vi "Configure.vi"(8 "error in (no error)":errorcluster, 11 "StageSPIM in":refnum<class "StageSPIM.lvclass">) -> (0 "error out":errorcluster, 2 "cancelled?":bool, 3 "StageSPIM out":refnum<class "StageSPIM.lvclass">)   [LabVIEW 2012, in "StageSPIM.lvclass"]
doc: "The configure method configures the details for the RabbitMQ connection. \n\nIn the derived class, make a call to the parent for setting these parameters."
uses:
  StageSPIM.lvclass
  connection_type.ctl
  baud_rate_control.ctl
  port_control.ctl
  <vilib>/Utility/miscctls.llb/LVPointTypeDef.ctl
  StageSPIM.lvclass/StageSPIM.ctl
  <vilib>/Distrio/Murmex/Murmex/Murmex.lvclass
panel:
  in  "button::configure murmex":bool
  in  "button::ok":bool
  in  "button::cancel":bool
  in  "Tab Control":enum32{"Comport", "Stages", "Debug"}(tab)
  in  "Port":T1 items=["COM1", "COM2", "COM3", "COM4", "COM5", "COM6", "COM7", "COM8", "COM9", "COM10", "COM11", "COM12", "COM13", "COM14", "COM15", "COM16", "COM17", "COM18", "COM19", "COM20", "COM21", "COM22", "COM23", "COM24", "COM25", "COM26", "COM27", "COM28", "COM29", "COM30"]
  in  "Baudrate":T2=3 items=["9600", "14400", "19200", "38400", "57600", "115200"]
  in  "Interface":T3=enum."USB_DaisyChain"
  in  "S/N Master controller":string
  in  "Update frequency":dbl[unit]
  in  "speedFocus":dbl[unit]
  in  "speedZ":dbl[unit]
  in  "speedY":dbl[unit]
  in  "speedX":dbl[unit]
  in  "soft min limit":dbl[](array[numeric])
  in  "soft max limit":dbl[](array[numeric])
  # "startup speed"
  # "X"
  # "Y"
  # "Z"
  # "Focus"
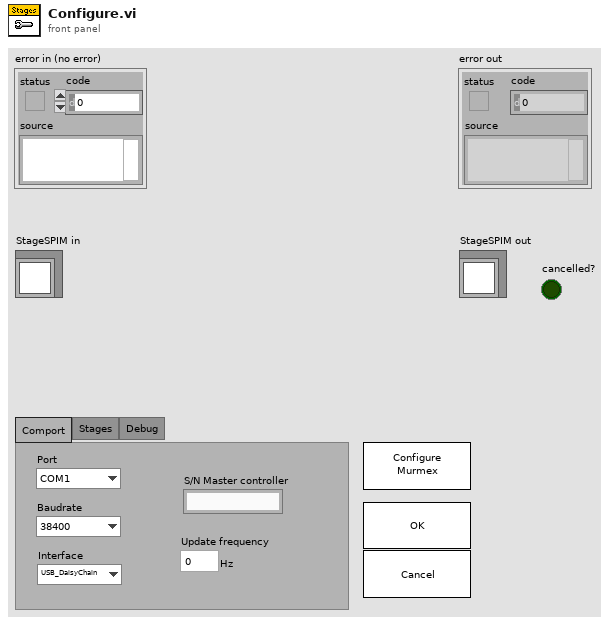
[diagram p1: front panel]
types:
  T1 = typedef "StageSPIM.lvclass/port_control.ctl" = i32
  T2 = typedef "StageSPIM.lvclass/baud_rate_control.ctl" = u16
  T3 = typedef "StageSPIM.lvclass/connection_type.ctl" = enum16{"RS232", "RS232 DaisyChain", "USB", "USB_DaisyChain"}
  T4 = typedef "LVPointTypeDef.ctl" = cluster{"Horizontal":i16, "Vertical":i16}
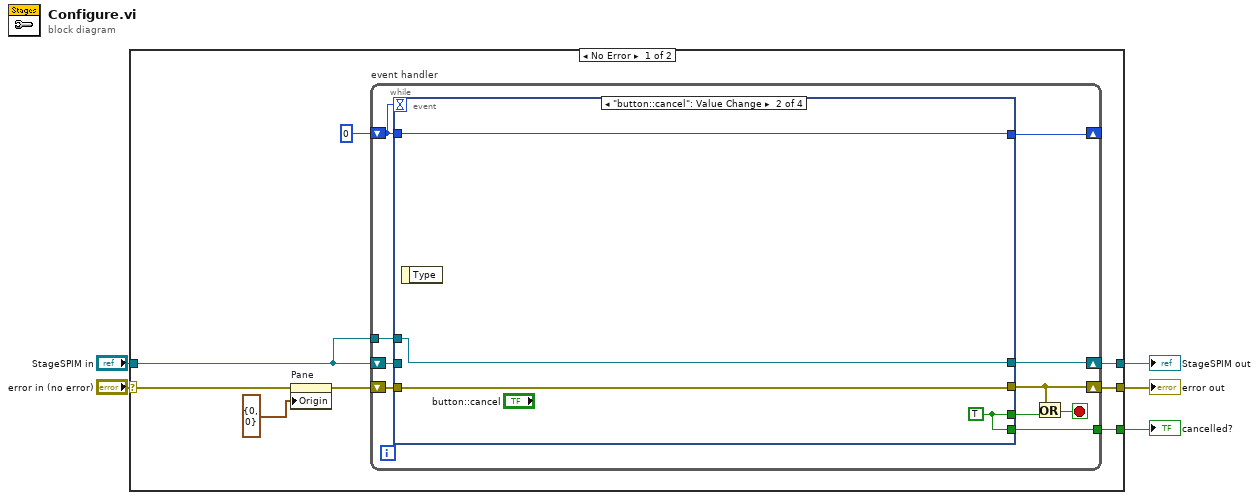
[diagram p0: block diagram]
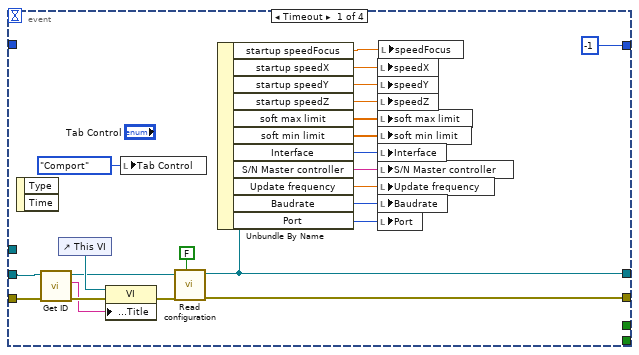
[diagram p2: hidden frame]
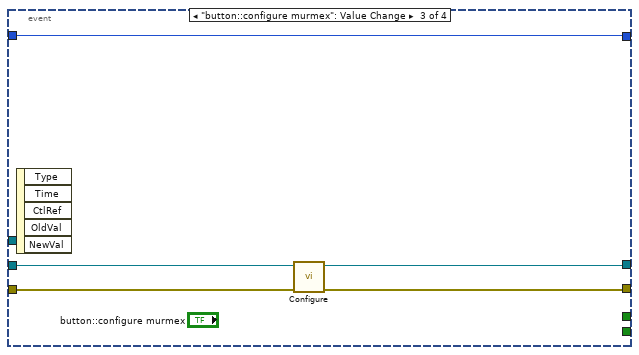
[diagram p3: hidden frame]
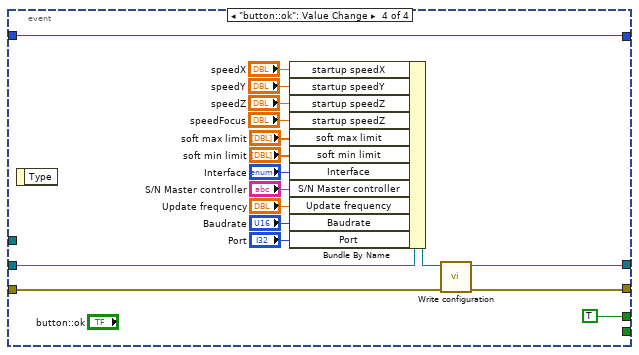
[diagram p4: hidden frame]
diagram:
  n1 = case shown="No Error" "error in (no error)" {
    selector: "error in (no error)" -> [w13 w74]
    tunnel: "StageSPIM in" -> [w10 w75]
    tunnel: [w8 w74] -> w3
    tunnel: [w7 w75] -> w2
    tunnel: [w6 _] -> w1
    frame No Error {
      n2 = property on="Pane" class="Pane"(error in=w13, "Origin"=T4 {"Horizontal"=0, "Vertical"=0}) -> (error out=w9:errorcluster)  [unwired: 1 in, 1 out]
      n3 = while "event handler" {
        shift-right: [w18] -> _
        shift-left: 0 -> [w23]
        shift-right: [w19] -> w7
        shift-left: w10 -> [w22]
        tunnel: w10 -> [w21]
        shift-right: [w16] -> w8
        shift-left: w9 -> [w20]
        tunnel: [w14] -> w6
        stop <- w17 stop-if-true
        n4 = event shown="[1] \"button::cancel\": Value Change" {
          selector: _ -> [_ _ _ _]
          dyn-events: _ -> [_ _ _ _]
          timeout: w23 -> [_ _ _ _]
          tunnel: w23 -> [_ w47 w51 w67]
          tunnel: w22 -> [w42 _ w53 w71]
          tunnel: w21 -> [_ w48 _ _]
          tunnel: w20 -> [w46 w50 w55 w73]
          tunnel: [w37 w48 w52 w69] -> w19
          tunnel: [w38 w50 w54 w72] -> w16
          tunnel: [-1 w47 w51 w67] -> w18
          tunnel: [_ w49 _ TRUE ("force loading?")] -> w15
          tunnel: [_ w49 _ _] -> w14
          event Timeout {
            n5 = event-data() -> ()  [unwired: 1 in, 2 out]
            n6 = call <vilib>:"Get ID.vi"("error in (no error)"=w46, "Murmex in"=w42) -> ("error out"=w45:errorcluster, "component id"=w43:string, "Murmex out"=w40:refnum<class "StageSPIM.lvclass">)  [unwired: 7 in]
            n7 = control-ref of="This VI"() -> (w44:refnum<vi>)
            n8 = property class="VI"(reference=w44, error in=w45, "Front Panel.Title"=w43) -> (error out=w41:errorcluster)  [unwired: 1 out]
            n9 = local write "Tab Control"(enum32{"Comport", "Stages", "Debug"}."Comport" ("Tab Control")) -> ()
            n10 = call-dynamic "Read configuration.vi"("force loading?"=FALSE, "error in (no error)"=w41, "StageSPIM in"=w40) -> ("error out"=w38:errorcluster, "StageSPIM out"=w37:refnum<class "StageSPIM.lvclass">)  [unwired: 7 in]
            n11 = Unbundle By Name(w37) -> ("startup speedFocus"=w24:dbl[unit], "startup speedX"=w27:dbl[unit], "startup speedY"=w26:dbl[unit], "startup speedZ"=w25:dbl[unit], "soft max limit"=w35:dbl[], "soft min limit"=w34:dbl[], "Interface"=w33:T3, "S/N Master controller"=w32:string, "Update frequency"=w31:dbl[unit], "Baudrate"=w30:T2, "Port"=w29:T1)
            n12 = local write "speedX"(w27) -> ()
            n13 = local write "speedY"(w26) -> ()
            n14 = local write "speedZ"(w25) -> ()
            n15 = local write "soft max limit"(w35) -> ()
            n16 = local write "soft min limit"(w34) -> ()
            n17 = local write "Interface"(w33) -> ()
            n18 = local write "S/N Master controller"(w32) -> ()
            n19 = local write "Update frequency"(w31) -> ()
            n20 = local write "Baudrate"(w30) -> ()
            n21 = local write "Port"(w29) -> ()
            n22 = local write "speedFocus"(w24) -> ()
          }
          event "button::cancel": Value Change {
            w49 = TRUE ("force loading?")
            n23 = event-data() -> ()  [unwired: 1 in, 1 out]
          }
          event "button::configure murmex": Value Change {
            n24 = event-data() -> ()  [unwired: 1 in, 5 out]
            n25 = call-parent "Configure.vi"("error in (no error)"=w55, "Murmex in"=w53) -> ("error out"=w54:errorcluster, "Murmex out"=w52:refnum<class "StageSPIM.lvclass">)  [unwired: 7 in, 1 out]
          }
          event "button::ok": Value Change {
            n26 = event-data() -> ()  [unwired: 1 in, 1 out]
            n27 = Bundle By Name(cluster=w71, "startup speedX"="speedX", "startup speedY"="speedY", "startup speedZ"="speedZ", "startup speedZ"="speedFocus", "soft max limit"="soft max limit", "soft min limit"="soft min limit", "Interface"="Interface", "S/N Master controller"="S/N Master controller", "Update frequency"="Update frequency", "Baudrate"="Baudrate", "Port"="Port") -> (w70:refnum<class "StageSPIM.lvclass">)
            n28 = call-dynamic "Write configuration.vi"("error in (no error)"=w73, "StageSPIM in"=w70) -> ("error out"=w72:errorcluster, "StageSPIM out"=w69:refnum<class "StageSPIM.lvclass">)  [unwired: 8 in]
          }
        }
        n29 = Or(x=w16, y=w15) -> (x .or. y?=w17:bool)
      }
    }
    frame Error {
    }
  }
  "error out" <- w3
  "StageSPIM out" <- w2
  "cancelled?" <- w1
